vi "Initial AIO Parameters.vi"(10 "Compiled.Settings":T5={"Name"="", "AO Enable"=FALSE, "AI Enable"=FALSE, "Main Page Parameters"={"AI Channels Used"=0, "AO Channels Used"=0, "Select channel type to add"="", "Device Name in Max"="PXI1Slot2", "PCL Decimation"=0, "Async Timeout (ms)"=0}, "Output Channel Parameters"={"AO MaxV"=0.0, "AO MinV"=0.0}, "AI Signals properties Array"=[], "AI Sample Rate"=0.0, "PCL Rate [Hz]"=0.0} {"AI Signals properties Array"."Input Configuration" items=["RSE"=10083, "NRSE"=10078, "Differential"=10106]}) -> (1 "AO Properties":T1, 3 "AI Properties":T3 {"AI Signals properties Array"."Input Configuration" items=["RSE"=10083, "NRSE"=10078, "Differential"=10106]})   [LabVIEW 2021, in "DAQ Analog InOut Engine.lvlib"]
uses:
  DAQ Analog InOut Engine.lvlib
  Shared/Compiled.Settings.ctl
  System Explorer/Types/Output Channel Parameters.ctl
  System Explorer/Types/Input Channel Parameters.ctl
  AI Properties.ctl
  AO Properties.ctl
  System Explorer/DAQ Analog InOut System Explorer.lvlib
  Shared/DAQ Analog InOut Shared.lvlib
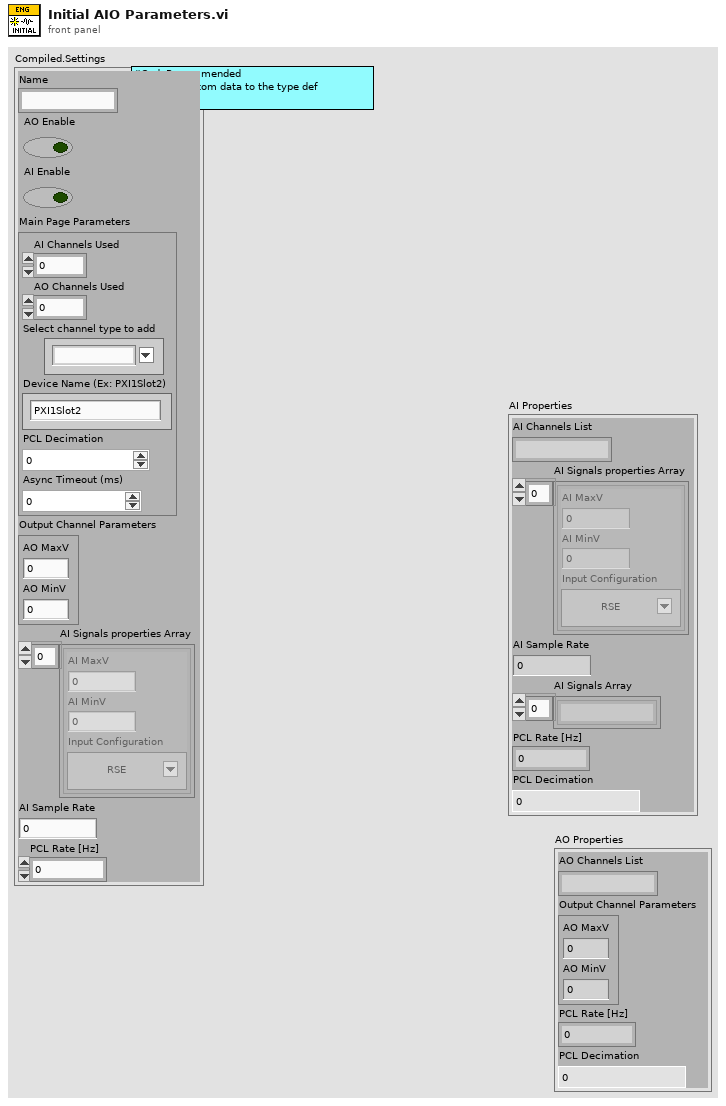
[diagram p1: front panel]
types:
  T1 = typedef "DAQ Analog InOut Engine.lvlib/AO Properties.ctl" = cluster{"AO Channels List":string, "Output Channel Parameters":T2, "PCL Rate [Hz]":dbl, "PCL Decimation":u16}
  T2 = typedef "DAQ Analog InOut System Explorer.lvlib/Output Channel Parameters.ctl" = cluster{"AO MaxV":dbl, "AO MinV":dbl}
  T3 = typedef "DAQ Analog InOut Engine.lvlib/AI Properties.ctl" = cluster{"AI Channels List":string, "AI Signals properties Array":T4[], "AI Sample Rate":dbl, "AI Signals Array":string[], "PCL Rate [Hz]":dbl, "PCL Decimation":u16}
  T4 = typedef "DAQ Analog InOut System Explorer.lvlib/Input Channel Parameters.ctl" = cluster{"AI MaxV":dbl, "AI MinV":dbl, "Input Configuration":u16}
  T5 = typedef "DAQ Analog InOut Shared.lvlib/Compiled.Settings.ctl" = cluster{"Name":string, "AO Enable":bool, "AI Enable":bool, "Main Page Parameters":cluster{"AI Channels Used":u8, "AO Channels Used":u8, "Select channel type to add":string, "Device Name in Max":string, "PCL Decimation":u16, "Async Timeout (ms)":u16}, "Output Channel Parameters":T2, "AI Signals properties Array":T4[], "AI Sample Rate":dbl, "PCL Rate [Hz]":dbl}
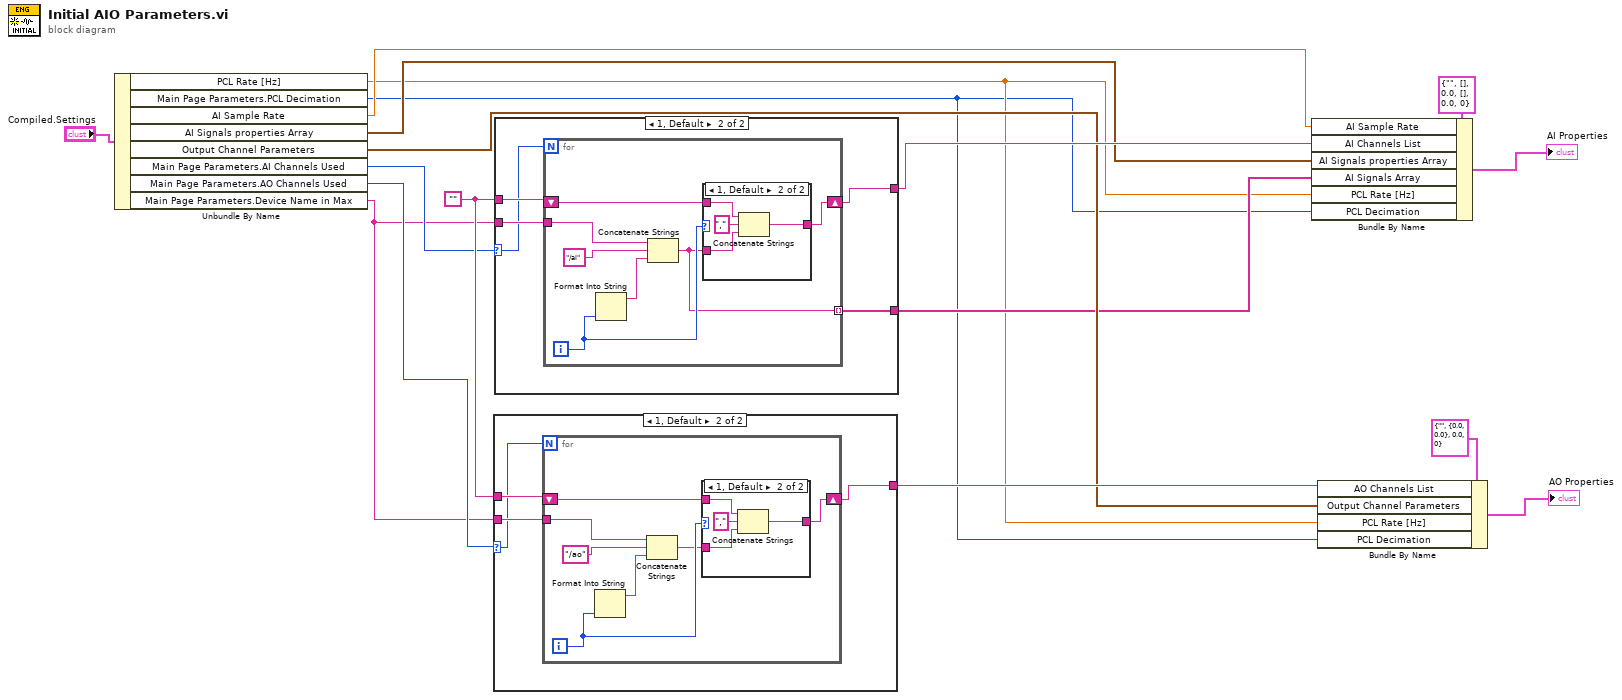
[diagram p0: block diagram]
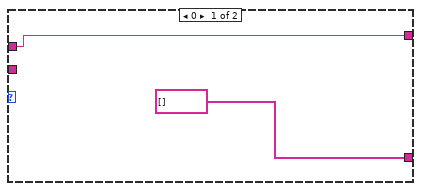
[diagram p4: hidden frame]
diagram:
  w17 = ""
  n1 = Unbundle By Name("Compiled.Settings") -> ("PCL Rate [Hz]"=w2:dbl, "Main Page Parameters.PCL Decimation"=w1:u16, "AI Sample Rate"=w4:dbl, "AI Signals properties Array"=w10:T4[], "Output Channel Parameters"=w7:T2, "Main Page Parameters.AI Channels Used"=w15:u8, "Main Page Parameters.AO Channels Used"=w14:u8, "Main Page Parameters.Device Name in Max"=w13:string)
  n2 = case shown="1, Default" w14 {
    selector: w14 -> [_ w19]
    tunnel: w13 -> [_ w22]
    tunnel: w17 -> [w18 w21]
    tunnel: [w18 w20] -> w8
    frame 0 {
    }
    frame 1, Default {
      n3 = for {
        N: w19 -> [_]
        tunnel: w22 -> [w29]
        shift-right: [w23] -> w20
        shift-left: w21 -> [w24]
        i -> [w26]
        n4 = Format Into String(w26) -> (resulting string=w27:string)  [unwired: 3 in, 1 out]
        n5 = Concatenate Strings(w29, "/ao", w27) -> (w25:string)
        n6 = case shown="1, Default" w26 {
          tunnel: w25 -> [w30 w34]
          tunnel: w24 -> [_ w32]
          tunnel: [w30 w31] -> w23
          frame 0 {
          }
          frame 1, Default {
            n7 = Concatenate Strings(w32, "," ("string"), w34) -> (w31:string)
          }
        }
      }
    }
  }
  n8 = case shown="1, Default" w15 {
    selector: w15 -> [_ w38]
    tunnel: w13 -> [_ w41]
    tunnel: w17 -> [w36 w40]
    tunnel: [w36 w39] -> w11
    tunnel: [string[] [] w37] -> w3
    frame 0 {
    }
    frame 1, Default {
      n9 = for {
        N: w38 -> [_]
        tunnel: w41 -> [w48]
        shift-right: [w43] -> w39
        shift-left: w40 -> [w44]
        tunnel: [w42] -> w37 mode=indexing
        i -> [w45]
        n10 = Format Into String(w45) -> (resulting string=w46:string)  [unwired: 3 in, 1 out]
        n11 = Concatenate Strings(w48, "/ai", w46) -> (w42:string)
        n12 = case shown="1, Default" w45 {
          tunnel: w42 -> [w49 w53]
          tunnel: w44 -> [_ w51]
          tunnel: [w49 w50] -> w43
          frame 0 {
          }
          frame 1, Default {
            n13 = Concatenate Strings(w51, "," ("string"), w53) -> (w50:string)
          }
        }
      }
    }
  }
  n14 = Bundle By Name(cluster=T3 {"AI Channels List"="", "AI Signals properties Array"=[], "AI Sample Rate"=0.0, "AI Signals Array"=[], "PCL Rate [Hz]"=0.0, "PCL Decimation"=0} ("AI Properties"), "AI Sample Rate"=w4, "AI Channels List"=w11, "AI Signals properties Array"=w10, "AI Signals Array"=w3, "PCL Rate [Hz]"=w2, "PCL Decimation"=w1) -> (→"AI Properties":T3)
  n15 = Bundle By Name(cluster=T1 {"AO Channels List"="", "Output Channel Parameters"={"AO MaxV"=0.0, "AO MinV"=0.0}, "PCL Rate [Hz]"=0.0, "PCL Decimation"=0} ("AO Properties"), "AO Channels List"=w8, "Output Channel Parameters"=w7, "PCL Rate [Hz]"=w2, "PCL Decimation"=w1) -> (→"AO Properties":T1)
